vi "WPI_CompressorClose.vi"(8 "error in (no error)":errorcluster, 11 "CompressorDevRef":T1) -> (0 "error out":errorcluster)   [LabVIEW 2017]
doc: "Closes the reference to the compressor you specify. Use this VI to close each compressor reference that you open with the Open VI. If you do not stop a running compressor with the Stop VI, closing the reference to the compressor stops the compressor.\n\nThis software is licensed. Open the labview\\readme\\WPI Robotics Library Open Source License.txt file for more information."
uses:
  <vilib>/Rock Robotics/WPI/Compressor/WPI_CompressorDevRef.ctl
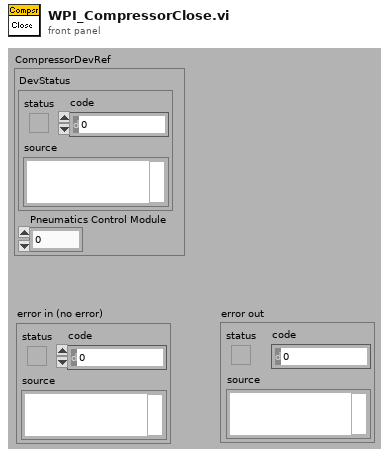
[diagram p1: front panel]
types:
  T1 = typedef "WPI_CompressorDevRef.ctl" = cluster{"DevStatus":errorcluster, "Pneumatics Control Module":u8}
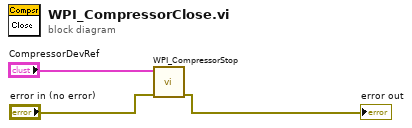
[diagram p0: block diagram]
diagram:
  n1 = call <vilib>:"WPI_CompressorStop.vi"("error in (no error)"="error in (no error)", "CompressorDevRef"="CompressorDevRef") -> ("error out"=→"error out":errorcluster)  [unwired: 9 out]
